vi "TPP-printer-v3.3.vi"() -> ()   [LabVIEW 2015]
uses:
  <vilib>/Math Plots/3D Math Plots/3D Scatter/3D Scatter XCtrl/3D Scatter.xctl
  <vilib>/DAQmx/write.llb/DAQmx Write (Digital Bool 1Line 1Point).vi
  SubNPC3SG.llb/device variables.vi
  <vilib>/Utility/file.llb/Read Delimited Spreadsheet (I64).vi
  <vilib>/Math Plots/3D Math Plots/3D Scatter/3D Scatter Datatype/Public/Plot Helper (Vector).vi
  <vilib>/DAQmx/create/channels.llb/DAQmx Create Channel (DO-Digital Output).vi
  <vilib>/DAQmx/miscellaneous.llb/DAQmx Fill In Error Info.vi
  <vilib>/Math Plots/3D Math Plots/3D Scatter/3D Scatter Datatype/3D Scatter Datatype.lvclass
panel:
  in  "Stopp":bool
  in  "Z轴驱动序列号":string="27002049"
  out "当前状态：":string
  in  "选项卡控件":enum32{"参数设置", "模型预览", "打印监控", "信息反馈"}(tab)
  in  "打印设置":T1={"f_objecitve(mm)"=1.8, "f_tubelens(mm)"=200.0, "f_scanlens(mm)"=50.0, "模型高/um"=2.0, "XY速度(um/s) "=0.0, "比例因子(V/°)"=1.0}
  in  "I/O 设置":T2={"matlab函数目录"=path "C:/Users/eason/Documents/GitHub/TPP-3D-printer/Matlab", "读取点阵文件"=path "C:/Users/eason/Documents/GitHub/TPP-3D-printer/Matlab/grating.txt", "DO通道：shutter控制"="Dev1/port1/line0", "AO通道：X前Y后"="Dev1/ao0:1", "Z轴驱动序列号"="27002049"}
  in  "刷新设置":bool
  out "三维散点图":refnum<class "3D Plot Datatype.lvclass">[](xcontrol)
  in  "取消打印":bool
  in  "开始打印":bool
  out "XYZG当前值/um":dbl[](array[numeric])=[-6.2105263157894735, -0.5263157894736842, 0.0, 1.0] format="%#.2g"
  out "每点耗时/ms":dbl=12.012958526611328 format="%#.0f"
  out "每行耗时/s":dbl=1.5567584037780762 format="%#.2g"
  out "每层耗时/min":dbl format="%#.2g"
  out "当前完成量：":u8(slide)=3 scale=0.0..100.0
  out "%":dbl=3.284878476249388 format="%#.2g"
  out "耗时/min":dbl=1.0008915185928344 format="%#.2g"
  in  "选项卡控件 2":enum32{"路径模拟", "PZT监控"}(tab)
  out "三维散点图 2":refnum<class "3D Plot Datatype.lvclass">[](xcontrol)
  in  "Drehschalter 2":dbl(knob) caption="2" min=-10.0 max=90.0 scale=0.0..100.0 scale format="%.3f"
  in  "Drehschalter 1":dbl(knob) caption="1" min=-10.0 max=90.0 scale=0.0..100.0 scale format="%.3f"
  in  "Drehschalter 0":dbl(knob) caption="0" min=-10.0 max=90.0 scale=0.0..100.0 scale format="%.3f"
  in  "Registerkarte":T3(tab)
  in  "Loop 2":bool caption="Loop"
  in  "Remote 2":bool caption="Remote"
  in  "Loop 1":bool caption="Loop"
  in  "Remote 1":bool caption="Remote"
  in  "Remote 0":bool caption="Remote"
  in  "Loop 0":bool caption="Loop"
  in  "Port":refnum<visa-resource-name>="COM1"
  in  "Refresh":bool
  out "Serial Number":string="RS232"
  out "Firmware Release Date":string="RS232"
  out "Version Number":string="RS232"
  out "Device":string="RS232"
  in  "com-write":bool caption="Logging"
  out "Receive Buffer":string
  out "Send Buffer":string
  in  "SendString":string caption="Enter Command"
  in  "Send":bool caption="Temp"
  in  "Clear":bool caption="Temp"
  out "Last Error":string="RS232"
  out "Last Command":string="RS232" caption="Command"
  in  "save sequence":bool caption="Loop"
  in  "load sequence":bool caption="Loop"
  in  "start sequence":bool caption="Loop"
  in  "sequence string":string
  out "时刻":T4={"点时间"=timestamp(3595558893.17812 s since 1904-01-01), "行时间"=timestamp(3595558891.757594 s since 1904-01-01), "层时间"=timestamp(3595558833.124629 s since 1904-01-01)}
  out "起始时间":timestamp
  out "暂停时间/min":dbl=1.0008915185928344 format="%#.2g"
  out "当前扫描速度(um/s)":dbl
  in  "dc level 3 out":refnum<vi>
  in  "dc level 2 out":refnum<vi>
  in  "dc level 1 out":refnum<vi>
  in  "dc level 1 in":refnum<vi>
  in  "dc level 2 in":refnum<vi>
  in  "dc level 3 in":refnum<vi>
  in  "loop 1 in":refnum<vi>
  in  "loop 2 in":refnum<vi>
  in  "loop 3 in":refnum<vi>
  in  "command in":refnum<vi>
  out "XYZG坐标表":dbl[][](array[numeric])
  # "Piezo 1"
  # "Piezo 2"
  # "Piezo 3"
  # "Loop"
  # "Remote"
  # "possible commands in sequence\n\nset,1,2.34 (actuator position)\nwait,5  - (holding time in sec.)\nstop - (terminate sequence)\n\nexample:\nset,1,2.134\nwait,5\nset,0,22.66\nwait,10\nstop"
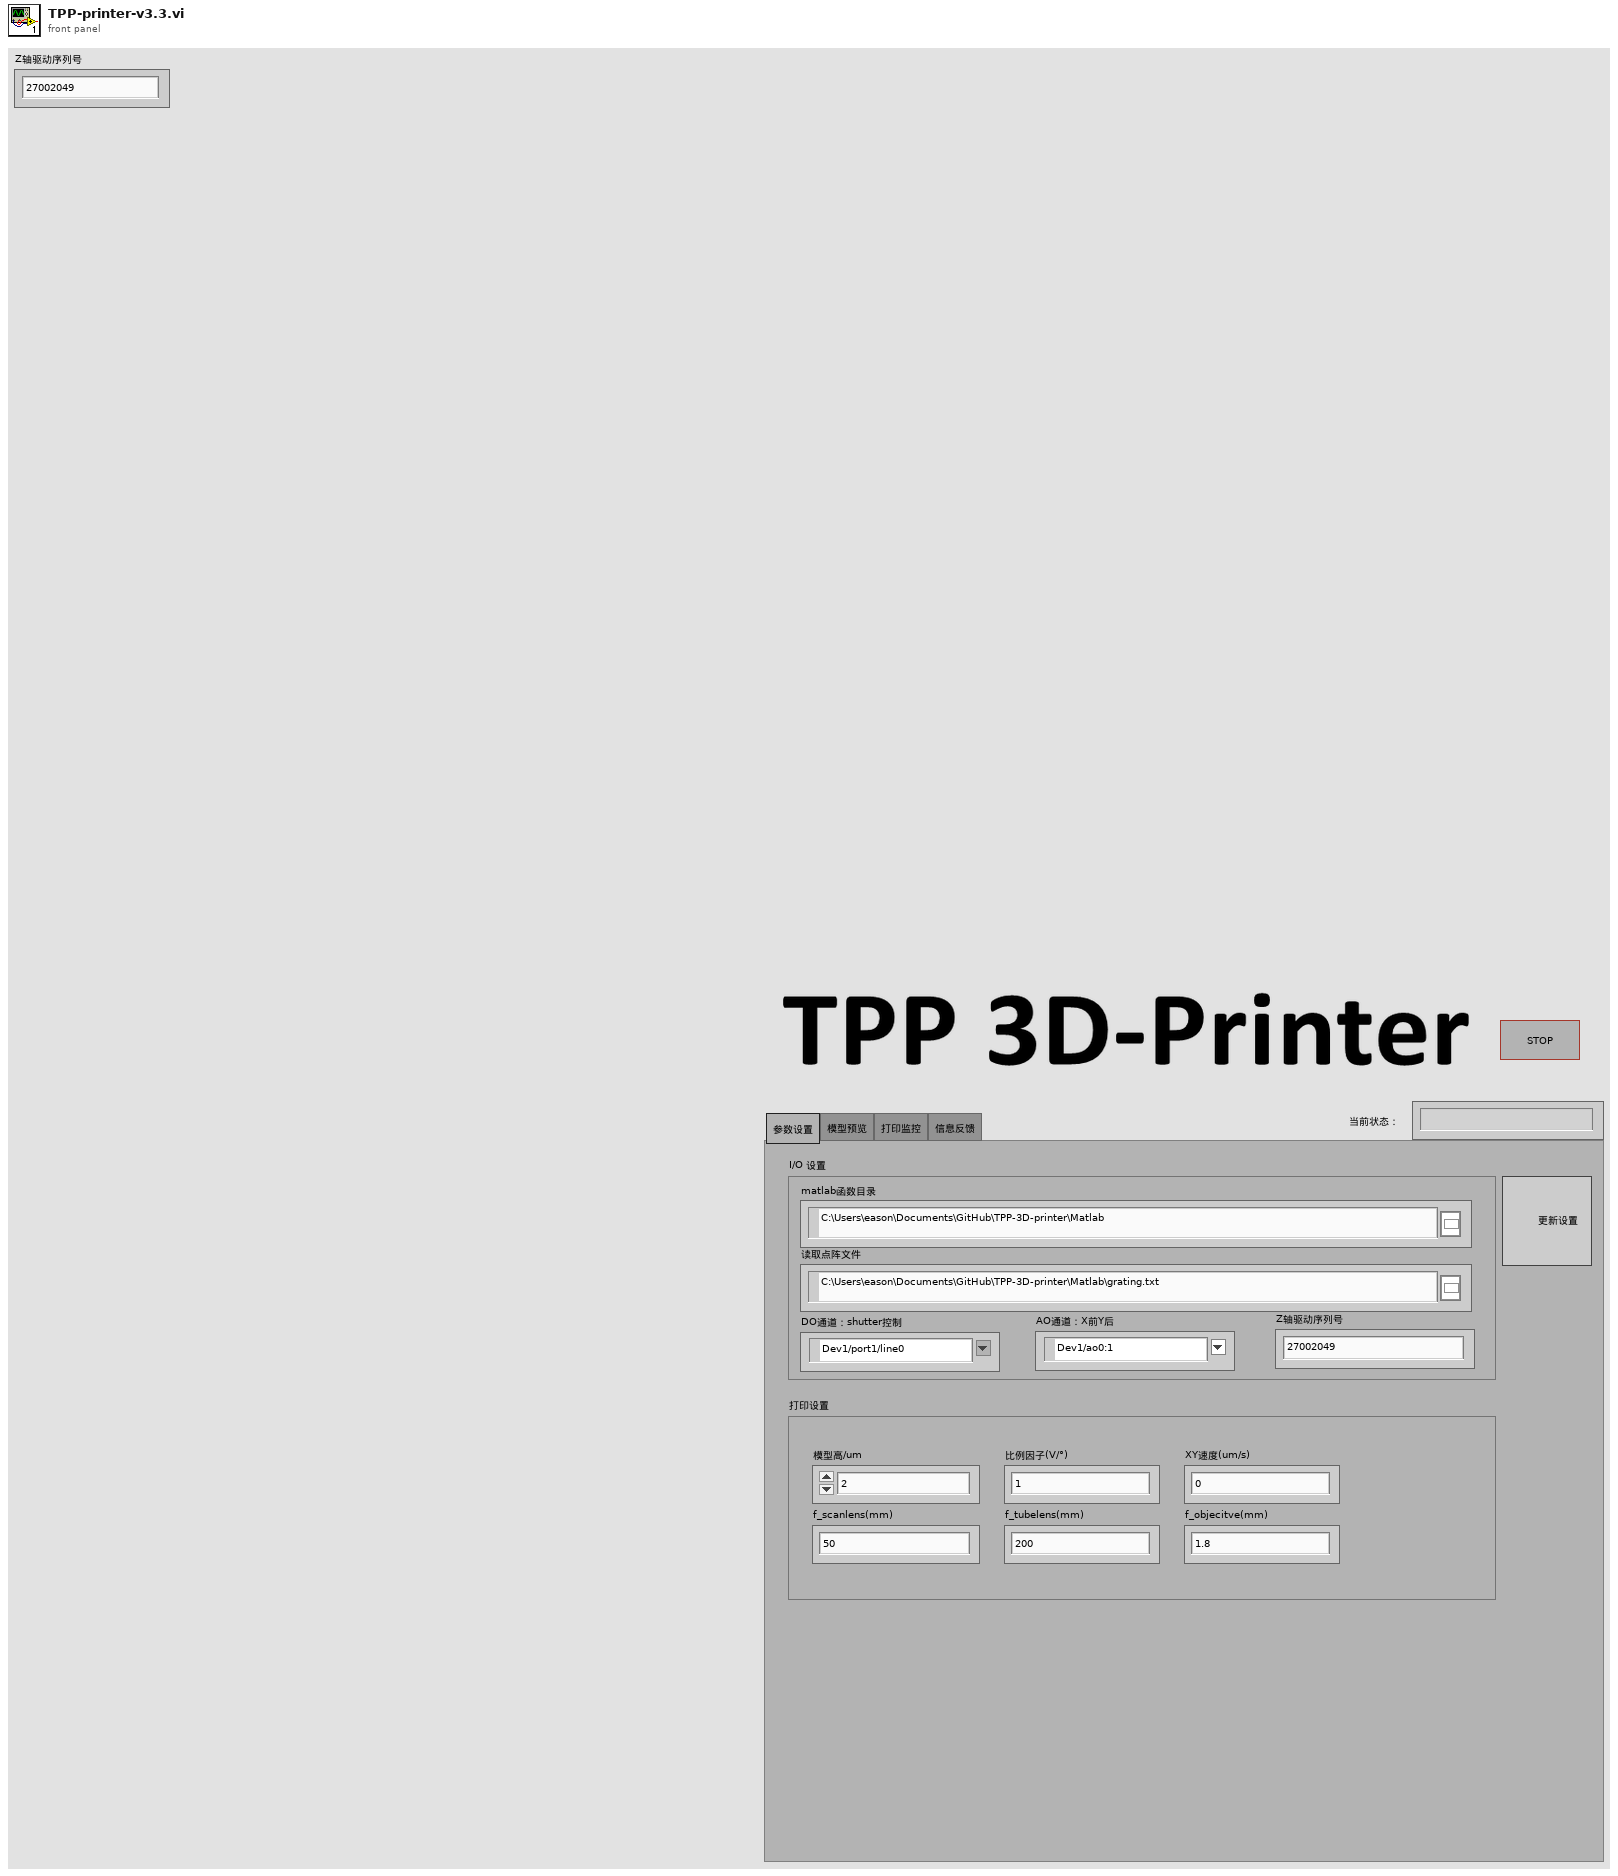
[diagram p1: front panel]
types:
  T1 = cluster{"f_objecitve(mm)":dbl, "f_tubelens(mm)":dbl, "f_scanlens(mm)":dbl, "模型高/um":dbl, "XY速度(um/s) ":dbl, "比例因子(V/°)":dbl}
  T2 = cluster{"matlab函数目录":path, "读取点阵文件":path, "DO通道：shutter控制":tag, "AO通道：X前Y后":tag, "Z轴驱动序列号":string}
  T3 = enum32{"Settings", "Info", "Communication", "Sequence"}
  T4 = cluster{"点时间":timestamp, "行时间":timestamp, "层时间":timestamp}
  T5 = enum16{"open", "replace", "create", "open or create", "replace or create", "replace or create with confirmation"}
  T6 = cluster{"Registerkarte":refnum<vi>, "Array IsActor":bool[], "Array loop":bool[], "Array remote":bool[]}
  T7 = cluster{"Array dc-level":dbl[], "VAR Temp":string, "VAR USB":string, "Array IsActor":bool[], "Array actor-name":string[], "Array axis":string[], "Array loop":bool[], "Array remote":bool[], "Array ovl":bool[]}
  T8 = cluster{"Drehschalter 0":refnum<vi>, "Drehschalter 1":refnum<vi>, "Drehschalter 2":refnum<vi>, "Array loop":bool[], "Array IsActor":bool[], "Array clmin":dbl[], "Array clmax":dbl[], "VAR Vmin":dbl, "VAR Vmax":dbl, "Array dc-level open":dbl[], "Array dc-level closed":dbl[], "VAR actualisation":bool}
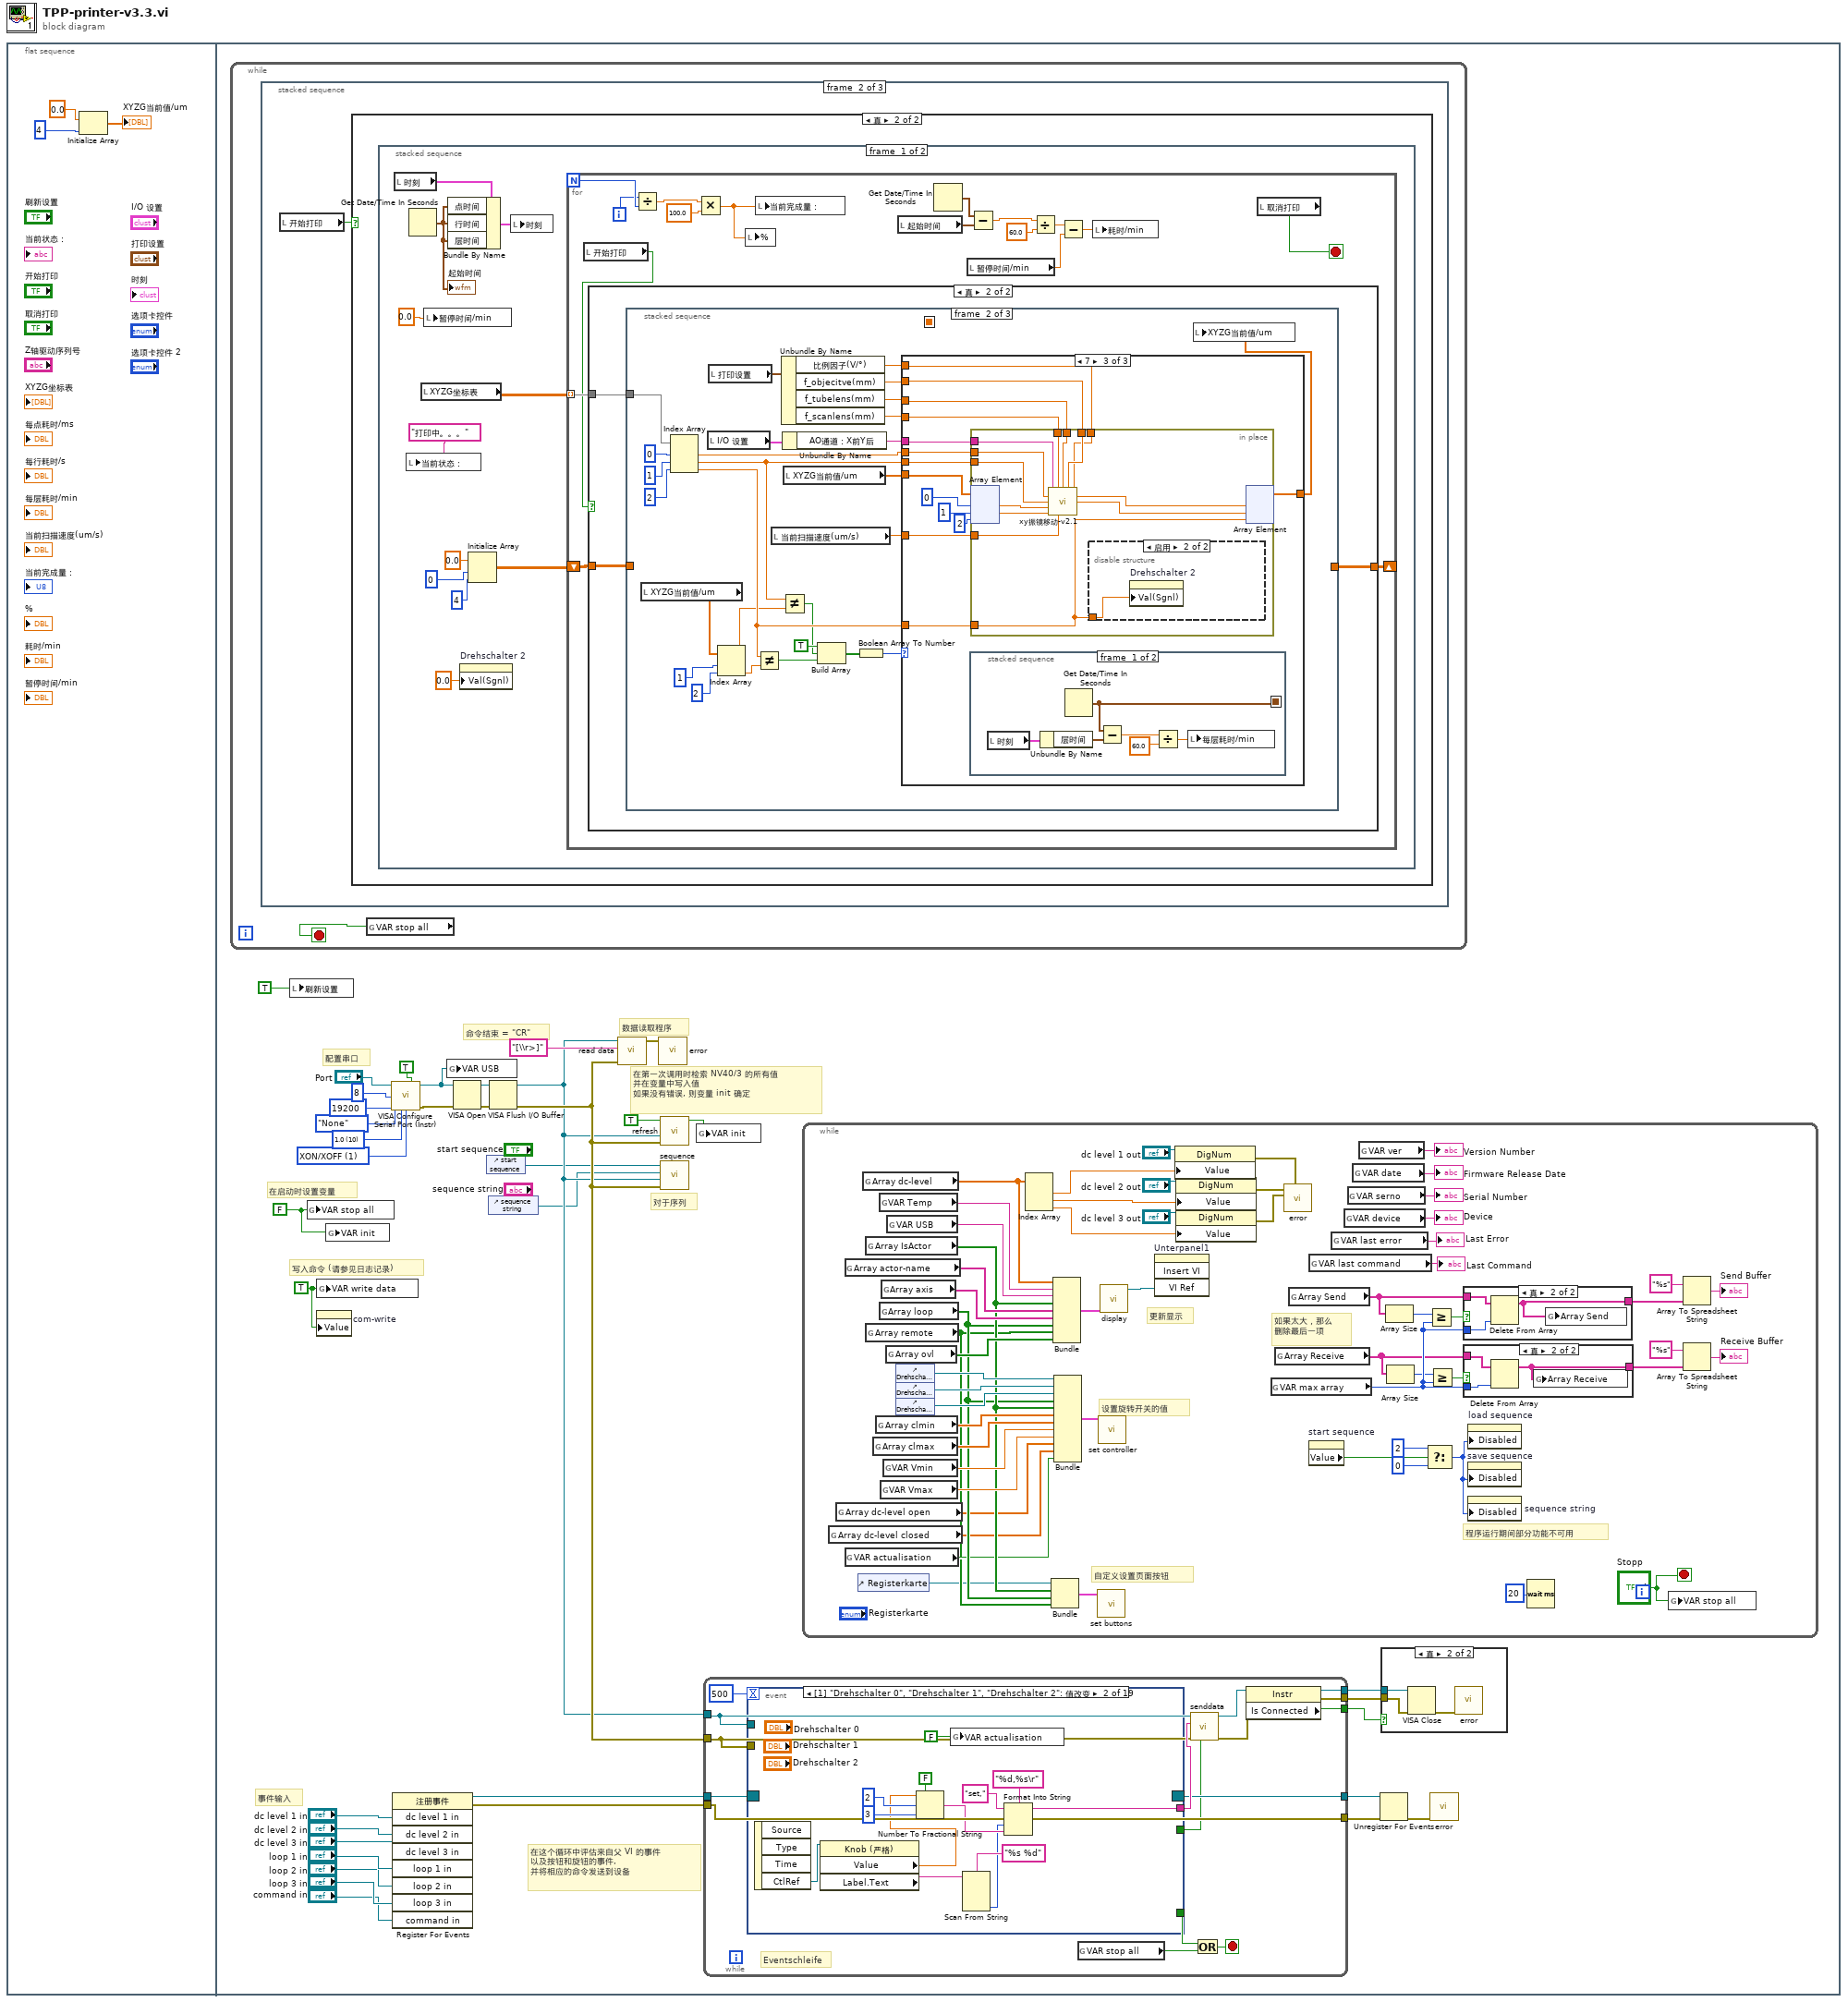
[diagram p0: block diagram]
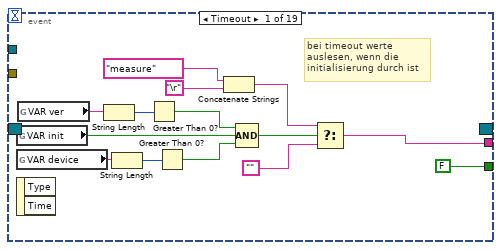
[diagram p3: hidden frame]
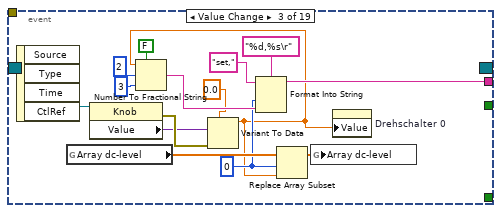
[diagram p4: hidden frame]
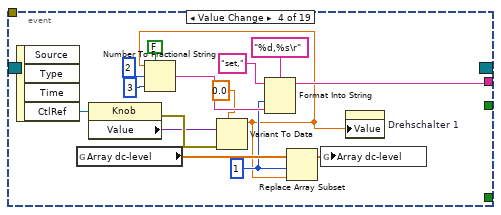
[diagram p5: hidden frame]
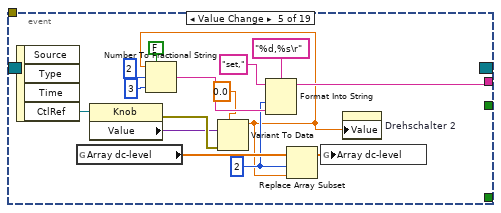
[diagram p6: hidden frame]
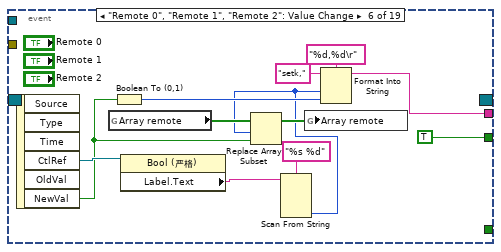
[diagram p7: hidden frame]
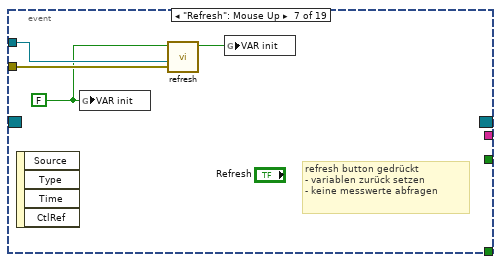
[diagram p8: hidden frame]
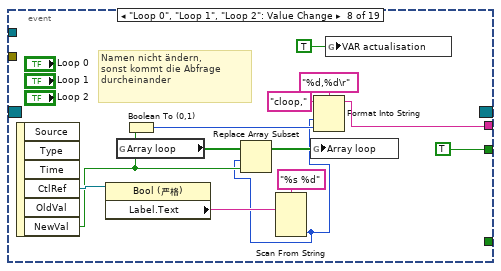
[diagram p9: hidden frame]
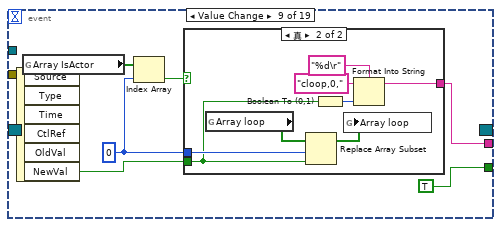
[diagram p10: hidden frame]
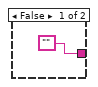
[diagram p11: hidden frame]
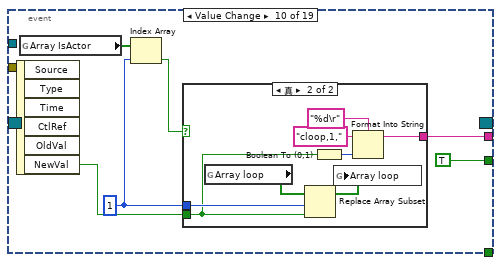
[diagram p12: hidden frame]
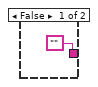
[diagram p13: hidden frame]
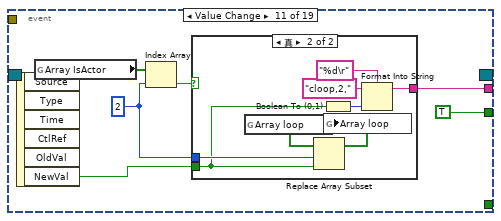
[diagram p14: hidden frame]
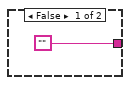
[diagram p15: hidden frame]
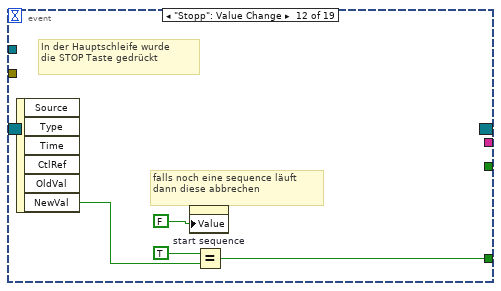
[diagram p16: hidden frame]
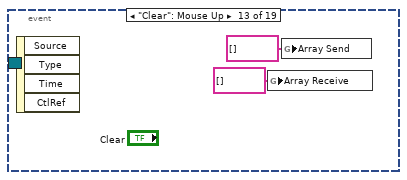
[diagram p17: hidden frame]
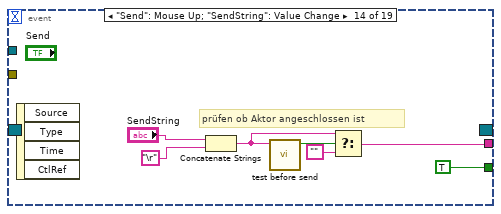
[diagram p18: hidden frame]
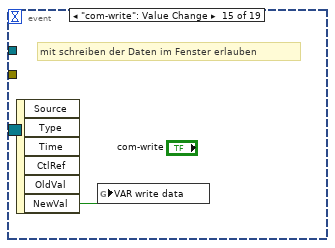
[diagram p19: hidden frame]
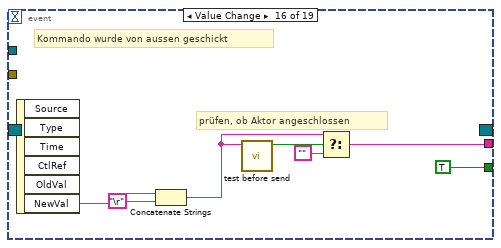
[diagram p20: hidden frame]
diagram:
  n1 = flat-sequence {
    frame #0 {
      n2 = Initialize Array(0.0 ("元素"), 4 ("维数大小")) -> (→"XYZG当前值/um":dbl[])
    }
    frame #1 {
      w12 = TRUE ("VAR write data")
      w16 = FALSE ("VAR ovl 3")
      w13 = u16 1 items=["Kein", "XON/XOFF", "RTS/CTS", "XON/XOFF & RTS/CTS", "DTR/DSR", "XON/XOFF & DTR/DSR"] ("flow control (0:none)")
      w32 = u16 10 items=["1.0"=10, "1.5"=15, "2.0"=20] ("stop bits (10: 1 bit)")
      # "对于序列"
      # "写入命令 (请参见日志记录)"
      # "命令结束 = \"CR\""
      # "数据读取程序"
      # "在第一次调用时检索 NV40/3 的所有值\n并在变量中写入值\n如果没有错误, 则变量 init 确定"
      # "在启动时设置变量"
      # "配置串口"
      # "事件输入"
      # "在这个循环中评估来自父 VI 的事件\n以及按钮和旋钮的事件, \n并将相应的命令发送到设备"
      n3 = while {
        stop <- w336 stop-if-true
        n4 = stacked-sequence {
          frame #0 {
            n5 = local read "刷新设置"() -> (w337:bool)
            n6 = case shown="真" w337 {
              frame False {
              }
              frame True {
                w344 = 0.0 ("每点耗时/ms")
                w353 = 0.0 ("速度(°/s)")
                # "平移坐标中心至X0Y0"
                n7 = local read "I/O 设置"() -> (w368:T2)
                n8 = local write "每点耗时/ms"(w344) -> ()
                n9 = local write "每行耗时/s"(w344) -> ()
                n10 = local write "每层耗时/min"(w344) -> ()
                n11 = disable-structure shown="禁用" {
                  disable-tunnel: w344 -> [w373 _]
                  frame Disabled {
                    n12 = local read "I/O 设置"() -> (w371:T2)
                    n13 = Unbundle By Name(w371) -> ("Z轴驱动序列号"=w370:string)
                    n14 = call "z物镜移动.vi"("position"=w373, "maxVelocity"=5.0, "SerialNumber"=w370) -> ()  [unwired: 6 in, 3 out]
                  }
                  frame Enabled {
                  }
                }
                n15 = Unbundle By Name(w368) -> ("matlab函数目录"=w366:path, "读取点阵文件"=w367:path)
                n16 = local read "打印设置"() -> (w365:T1)
                n17 = Unbundle By Name(w365) -> ("模型高/um"=w364:dbl)
                n18 = call-poly <vilib>:"Read Delimited Spreadsheet.vi"("file path (dialog if empty)"=w367) -> ("all rows"=w369:i64[][])  [unwired: 9 in, 5 out]
                n19 = script code="addpath(add_path);\ncol_x=2;\ncol_y=3;\ncol_z=4;\nxyzg=path_generation( in,col_x,col_y,col_z,z_length );"("in"=w369, "z_length"=w364, "add_path"=w366) -> ("xyzg"=w354:dbl[][])  [unwired: 1 in, 1 out]
                n20 = local read "打印设置"() -> (w350:T1)
                n21 = local read "I/O 设置"() -> (w352:T2)
                n22 = Unbundle By Name(w352) -> ("AO通道：X前Y后"=w351:tag)
                n23 = Unbundle By Name(w350) -> ("比例因子(V/°)"=w343:dbl, "f_objecitve(mm)"=w347:dbl, "f_tubelens(mm)"=w348:dbl, "f_scanlens(mm)"=w349:dbl)
                n24 = call "xy振镜移动-v2.1.vi"("AO通道：X前Y后"=w351, "f_scanlens(mm)"=w349, "f_tubelens(mm)"=w348, "f_objecitve(mm)"=w347, "比例因子(V/°)"=w343, "x终止位(um)"=w353, "y终止位(um)"=w353, "速度(um/s)"=w353) -> ()  [unwired: 6 in, 2 out]
                n25 = local write "XYZG坐标表"(w354) -> ()
                n26 = Array Max & Min(array=w354) -> (max value=w356:dbl, min value=w357:dbl)  [unwired: 2 out]
                n27 = Subtract(x=w356, y=w357) -> (x-y=w355:dbl)
                n28 = Index Array(array=w354, index (col) #1=0 ("禁用的索引 (列)"), index (col) #2=1 ("索引 (列)"), index (col) #3=2 ("索引 (列)")) -> (element #1=w360:dbl[], element #2=w359:dbl[], element #3=w358:dbl[])  [unwired: 3 in]
                n29 = local write "刷新设置"(FALSE ("刷新设置")) -> ()
                n30 = Divide(x=w360, y=w355) -> (x/y=w339:dbl[])
                n31 = Divide(x=w359, y=w355) -> (x/y=w338:dbl[])
                n32 = Divide(x=w358, y=w355) -> (x/y=w340:dbl[])
                n33 = local write "当前状态："("初始化。。。" ("当前状态：")) -> ()
                n34 = call-poly <vilib>:"Plot Helper.vi"("z vector"=w340, "y vector"=w338, "x vector"=w339) -> ("error out"=w341:errorcluster, "3D Plot lvclass Array out"=→"三维散点图":refnum<class "3D Plot Datatype.lvclass">[])  [unwired: 3 in, 4 out]
                n35 = call <vilib>:"Simple Error Handler.vi"("error in (no error)"=w341) -> ()  [unwired: 4 in, 5 out]
              }
            }
          }
          frame #1 {
            n36 = local read "开始打印"() -> (w374:bool)
            n37 = case shown="真" w374 {
              frame False {
              }
              frame True {
                n38 = stacked-sequence {
                  frame #0 {
                    n39 = local read "时刻"() -> (w382:T4)
                    n40 = local write "当前状态："("打印中。。。" ("当前状态：")) -> ()
                    n41 = Get Date/Time In Seconds() -> (seconds since 1Jan1904=w381:timestamp)
                    "起始时间" <- w381
                    n42 = local read "XYZG坐标表"() -> (w384:dbl[][])
                    n43 = local write "暂停时间/min"(0.0 ("暂停耗时/min")) -> ()
                    n44 = Bundle By Name(cluster=w382, "点时间"=w381, "行时间"=w381, "层时间"=w381) -> (w380:T4)
                    n45 = property on="Drehschalter 2" class="Knob (严格)"("Val(Sgnl)"=0.0 ("值(信号)")) -> ()  [unwired: 2 in, 2 out]
                    n46 = Initialize Array(0.0 ("元素"), 0 ("维数大小"), 4 ("维数大小")) -> (w378:dbl[][])
                    n47 = local write "时刻"(w380) -> ()
                    n48 = for {
                      N -> [w401]
                      tunnel: w384 -> [w402] mode=indexing
                      shift-right: [w387] -> _
                      shift-left: w378 -> [w388]
                      i -> [w386]
                      stop <- w397 stop-if-true
                      n49 = local read "开始打印"() -> (w398:bool)
                      n50 = case shown="真" w398 {
                        tunnel: w402 -> [_ w421]
                        tunnel: w388 -> [w403 w420]
                        tunnel: [w403 w419] -> w387
                        frame False {
                          n51 = stacked-sequence {
                            seq-local: [w404 _ _] -> [_ _ w412]
                            frame #0 {
                              n52 = Get Date/Time In Seconds() -> (seconds since 1Jan1904=w404:timestamp)
                            }
                            frame #1 {
                              n53 = while {
                                stop <- w406 stop-if-true
                                n54 = local read "开始打印"() -> (w408:bool)
                                n55 = local read "取消打印"() -> (w407:bool)
                                n56 = Or(x=w408, y=w407) -> (x .or. y?=w406:bool)
                              }
                              n57 = local write "当前状态："("暂停打印" ("当前状态：")) -> ()
                            }
                            frame #2 {
                              n58 = Get Date/Time In Seconds() -> (seconds since 1Jan1904=w409:timestamp)
                              n59 = local read "时刻"() -> (w411:T4)
                              n60 = Subtract(x=w409, y=w412) -> (x-y=w417:dbl)
                              n61 = Bundle By Name(cluster=w411, "点时间"=w409, "行时间"=w409, "层时间"=w409) -> (w410:T4)
                              n62 = local read "暂停时间/min"() -> (w414:dbl)
                              n63 = Divide(x=w417, y=60.0) -> (x/y=w415:dbl)
                              n64 = local write "时刻"(w410) -> ()
                              n65 = Add(x=w415, y=w414) -> (x+y=w413:dbl)
                              n66 = local write "暂停时间/min"(w413) -> ()
                              n67 = local write "当前状态："("打印中。。。" ("当前状态：")) -> ()
                            }
                          }
                        }
                        frame True {
                          n68 = stacked-sequence {
                            seq-local: [w423 _ _] -> [_ _ w595]
                            tunnel: w421 -> [w422 w469 _]
                            tunnel: w420 -> [_ _ w594]
                            tunnel: [_ _ w592] -> w419
                            frame #0 {
                              n69 = local read "XYZG当前值/um"() -> (w426:dbl[])
                              n70 = Index Array(array=w426, index=3 ("索引")) -> (element=w424:dbl)
                              n71 = Index Array(array=w422, index=3 ("禁用的索引 (列)")) -> (element=w423:dbl)
                              n72 = Not Equal?(x=w424, y=w423) -> (x != y?=w427:bool)
                              n73 = case shown="真" w427 {
                                tunnel: w423 -> [_ w430]
                                frame False {
                                }
                                frame True {
                                n74 = case shown="1" w430 {
                                frame 0, Default {
                                # "1，关闭shutter"
                                n75 = local read "I/O 设置"() -> (w434:T2)
                                n76 = Unbundle By Name(w434) -> ("DO通道：shutter控制"=w433:tag)
                                n77 = call-poly <vilib>:"DAQmx Create Virtual Channel.vi"("lines"=w433) -> ("task out"=w445:refnum<k21>, "error out"=w444:errorcluster)  [unwired: 13 in]
                                n78 = local write "当前扫描速度(um/s)"(0.0 ("扫描速度(°/s)")) -> ()
                                n79 = call-poly <vilib>:"DAQmx Write.vi"("task/channels in"=w445, "data"=FALSE, "error in"=w444) -> ("task out"=w442:refnum<k21>, "error out"=w441:errorcluster)  [unwired: 10 in, 1 out]
                                n80 = call <vilib>:"DAQmx Start Task.vi"("task/channels in"=w442, "error in"=w441) -> ("task out"=w436:refnum<k21>, "error out"=w435:errorcluster)  [unwired: 12 in]
                                n81 = call <vilib>:"DAQmx Stop Task.vi"("task/channels in"=w436, "error in"=w435) -> ("task out"=w440:refnum<k21>, "error out"=w439:errorcluster)  [unwired: 12 in]
                                n82 = call <vilib>:"DAQmx Clear Task.vi"("task in"=w440, "error in"=w439) -> ("error out"=w438:errorcluster)  [unwired: 13 in]
                                n83 = call <vilib>:"Simple Error Handler.vi"("error in (no error)"=w438) -> ()  [unwired: 4 in, 5 out]
                                }
                                frame 1 {
                                # "1，打开shutter\n2，设定速度（斜率）\n3，等待"
                                n84 = stacked-sequence {
                                frame #0 {
                                n85 = local read "I/O 设置"() -> (w449:T2)
                                n86 = Unbundle By Name(w449) -> ("DO通道：shutter控制"=w448:tag)
                                n87 = call-poly <vilib>:"DAQmx Create Virtual Channel.vi"("lines"=w448) -> ("task out"=w459:refnum<k21>, "error out"=w458:errorcluster)  [unwired: 13 in]
                                n88 = call-poly <vilib>:"DAQmx Write.vi"("task/channels in"=w459, "data"=TRUE, "error in"=w458) -> ("task out"=w456:refnum<k21>, "error out"=w455:errorcluster)  [unwired: 10 in, 1 out]
                                n89 = call <vilib>:"DAQmx Start Task.vi"("task/channels in"=w456, "error in"=w455) -> ("task out"=w451:refnum<k21>, "error out"=w450:errorcluster)  [unwired: 12 in]
                                n90 = call <vilib>:"DAQmx Stop Task.vi"("task/channels in"=w451, "error in"=w450) -> ("task out"=w454:refnum<k21>, "error out"=w453:errorcluster)  [unwired: 12 in]
                                n91 = call <vilib>:"DAQmx Clear Task.vi"("task in"=w454, "error in"=w453) -> ("error out"=w452:errorcluster)  [unwired: 13 in]
                                n92 = call <vilib>:"Simple Error Handler.vi"("error in (no error)"=w452) -> ()  [unwired: 4 in, 5 out]
                                }
                                frame #1 {
                                n93 = Wait (ms)(milliseconds to wait=u32 0 ("等待时间（毫秒）")) -> ()  [unwired: 1 out]
                                }
                                }
                                n94 = local read "打印设置"() -> (w447:T1)
                                n95 = Unbundle By Name(w447) -> ("XY速度(um/s)"=w446:dbl)
                                n96 = local write "当前扫描速度(um/s)"(w446) -> ()
                                }
                                }
                                n97 = local read "XYZG当前值/um"() -> (w432:dbl[])
                                n98 = Replace Array Subset(array=w432, new element=w430, index=3 ("索引")) -> (w429:dbl[])
                                n99 = local write "XYZG当前值/um"(w429) -> ()
                                }
                              }
                            }
                            frame #1 {
                              n100 = local read "XYZG当前值/um"() -> (w477:dbl[])
                              n101 = Index Array(array=w469, index #1=0 ("禁用的索引 (列)"), index #2=1 ("索引"), index #3=2 ("索引")) -> (element #1=w481:dbl, element #2=w472:dbl, element #3=w476:dbl)
                              n102 = local read "I/O 设置"() -> (w463:T2)
                              n103 = local read "打印设置"() -> (w468:T1)
                              n104 = Index Array(array=w477, index #1=1 ("索引"), index #2=2 ("索引")) -> (element #1=w471:dbl, element #2=w473:dbl)
                              n105 = Not Equal?(x=w476, y=w473) -> (x != y?=w475:bool)
                              n106 = local read "当前扫描速度(um/s)"() -> (w486:dbl)
                              n107 = Not Equal?(x=w472, y=w471) -> (x != y?=w470:bool)
                              n108 = Unbundle By Name(w468) -> ("比例因子(V/°)"=w467:dbl, "f_objecitve(mm)"=w465:dbl, "f_tubelens(mm)"=w466:dbl, "f_scanlens(mm)"=w464:dbl)
                              n109 = Unbundle By Name(w463) -> ("AO通道：X前Y后"=w462:tag)
                              n110 = local read "XYZG当前值/um"() -> (w484:dbl[])
                              n111 = Build Array(TRUE ("元素"), w470, w475) -> (w483:bool[])
                              n112 = Boolean Array To Number(Boolean array=w483) -> (number=w461:u32)
                              n113 = case shown="7" w461 {
                                tunnel: w462 -> [w493 w525 w561]
                                tunnel: w481 -> [w495 w526 w560]
                                tunnel: w484 -> [w498 w527 w559]
                                tunnel: [w489 w520 w551] -> w485
                                tunnel: w486 -> [w494 w528 w558]
                                tunnel: w472 -> [_ w524 w557]
                                tunnel: w476 -> [_ _ w552]
                                tunnel: w464 -> [w492 w523 w556]
                                tunnel: w466 -> [w491 w522 w555]
                                tunnel: w465 -> [w490 w521 w554]
                                tunnel: w467 -> [w488 w519 w550]
                                frame 1, Default {
                                n114 = stacked-sequence {
                                seq-local: [w501 _] -> [_ w507]
                                frame #0 {
                                n115 = local read "时刻"() -> (w499:T4)
                                n116 = Unbundle By Name(w499) -> ("点时间"=w500:timestamp)
                                n117 = Get Date/Time In Seconds() -> (seconds since 1Jan1904=w501:timestamp)
                                n118 = Subtract(x=w501, y=w500) -> (x-y=w504:dbl)
                                n119 = Multiply(x=w504, y=1000.0) -> (x*y=w502:dbl)
                                n120 = local write "每点耗时/ms"(w502) -> ()
                                }
                                frame #1 {
                                n121 = local read "时刻"() -> (w505:T4)
                                n122 = Bundle By Name(cluster=w505, "点时间"=w507) -> (w506:T4)
                                n123 = local write "时刻"(w506) -> ()
                                }
                                }
                                n124 = in-place {
                                in-place-border: w495 -> [w513]
                                in-place-border: w494 -> [w518]
                                in-place-border: w493 -> [w517]
                                in-place-border: w492 -> [w516]
                                in-place-border: w491 -> [w515]
                                in-place-border: w490 -> [w514]
                                in-place-border: w488 -> [w508]
                                n125 = in-place-array #1(w498, 0, 1) -> (w512:dbl, w511:dbl)
                                n126 = call "xy振镜移动-v2.1.vi"("AO通道：X前Y后"=w517, "f_scanlens(mm)"=w516, "f_tubelens(mm)"=w515, "f_objecitve(mm)"=w514, "比例因子(V/°)"=w508, "x终止位(um)"=w513, "y终止位(um)"=w511, "x初始位(um)"=w512, "y初始位(um)"=w511, "速度(um/s)"=w518) -> ("x终止位(um) 2"=w510:dbl, "y终止位(um) 2"=w509:dbl)  [unwired: 4 in]
                                n127 = in-place-array #1(w510, w509) -> (w489:dbl[])  [unwired: 2 out]
                                }
                                }
                                frame 3 {
                                n128 = in-place {
                                in-place-border: w526 -> [w549]
                                in-place-border: w528 -> [w548]
                                in-place-border: w525 -> [w547]
                                in-place-border: w524 -> [w543]
                                in-place-border: w523 -> [w546]
                                in-place-border: w522 -> [w545]
                                in-place-border: w521 -> [w544]
                                in-place-border: w519 -> [w538]
                                n129 = in-place-array #2(w527, 0, 1) -> (w542:dbl, w541:dbl)
                                n130 = call "xy振镜移动-v2.1.vi"("AO通道：X前Y后"=w547, "f_scanlens(mm)"=w546, "f_tubelens(mm)"=w545, "f_objecitve(mm)"=w544, "比例因子(V/°)"=w538, "x终止位(um)"=w549, "y终止位(um)"=w543, "x初始位(um)"=w542, "y初始位(um)"=w541, "速度(um/s)"=w548) -> ("x终止位(um) 2"=w540:dbl, "y终止位(um) 2"=w539:dbl)  [unwired: 4 in]
                                n131 = in-place-array #2(w540, w539) -> (w520:dbl[])  [unwired: 2 out]
                                }
                                n132 = stacked-sequence {
                                seq-local: [w533 _] -> [_ w537]
                                frame #0 {
                                n133 = local read "时刻"() -> (w531:T4)
                                n134 = Unbundle By Name(w531) -> ("行时间"=w532:timestamp)
                                n135 = Get Date/Time In Seconds() -> (seconds since 1Jan1904=w533:timestamp)
                                n136 = Subtract(x=w533, y=w532) -> (x-y=w534:dbl)
                                n137 = local write "每行耗时/s"(w534) -> ()
                                }
                                frame #1 {
                                n138 = local read "时刻"() -> (w535:T4)
                                n139 = Bundle By Name(cluster=w535, "行时间"=w537) -> (w536:T4)
                                n140 = local write "时刻"(w536) -> ()
                                }
                                }
                                }
                                frame 7 {
                                n141 = stacked-sequence {
                                seq-local: [w569 _] -> [_ w572]
                                frame #0 {
                                n142 = local read "时刻"() -> (w564:T4)
                                n143 = Unbundle By Name(w564) -> ("层时间"=w565:timestamp)
                                n144 = Get Date/Time In Seconds() -> (seconds since 1Jan1904=w569:timestamp)
                                n145 = Subtract(x=w569, y=w565) -> (x-y=w568:dbl)
                                n146 = Divide(x=w568, y=60.0) -> (x/y=w566:dbl)
                                n147 = local write "每层耗时/min"(w566) -> ()
                                }
                                frame #1 {
                                n148 = local read "时刻"() -> (w571:T4)
                                n149 = Bundle By Name(cluster=w571, "层时间"=w572) -> (w570:T4)
                                n150 = local write "时刻"(w570) -> ()
                                }
                                }
                                n151 = in-place {
                                in-place-border: w560 -> [w584]
                                in-place-border: w558 -> [w575]
                                in-place-border: w561 -> [w585]
                                in-place-border: w557 -> [w583]
                                in-place-border: w556 -> [w578]
                                in-place-border: w555 -> [w577]
                                in-place-border: w554 -> [w576]
                                in-place-border: w552 -> [w573]
                                in-place-border: w550 -> [w574]
                                n152 = in-place-array #3(w559, 0, 1, 2) -> (w580:dbl, w579:dbl)  [unwired: 1 out]
                                n153 = call "xy振镜移动-v2.1.vi"("AO通道：X前Y后"=w585, "f_scanlens(mm)"=w578, "f_tubelens(mm)"=w577, "f_objecitve(mm)"=w576, "比例因子(V/°)"=w574, "x终止位(um)"=w584, "y终止位(um)"=w583, "x初始位(um)"=w580, "y初始位(um)"=w579, "速度(um/s)"=w575) -> ("x终止位(um) 2"=w582:dbl, "y终止位(um) 2"=w581:dbl)  [unwired: 4 in]
                                n154 = disable-structure shown="启用" {
                                disable-tunnel: w573 -> [w589 w590]
                                frame Disabled {
                                n155 = local read "I/O 设置"() -> (w587:T2)
                                n156 = Unbundle By Name(w587) -> ("Z轴驱动序列号"=w586:string)
                                n157 = call "z物镜移动.vi"("position"=w589, "maxVelocity"=5.0, "SerialNumber"=w586) -> ()  [unwired: 6 in, 3 out]
                                }
                                frame Enabled {
                                n158 = property on="Drehschalter 2" class="Knob (严格)"("Val(Sgnl)"=w590) -> ()  [unwired: 2 in, 2 out]
                                }
                                }
                                n159 = in-place-array #3(w582, w581, w573) -> (w551:dbl[])  [unwired: 3 out]
                                }
                                }
                              }
                              n160 = local write "XYZG当前值/um"(w485) -> ()
                            }
                            frame #2 {
                              n161 = local read "XYZG当前值/um"() -> (w593:dbl[])
                              n162 = local read "选项卡控件 2"() -> (w591:enum32{"路径模拟", "PZT监控"})
                              n163 = Insert Into Array(array=w594, new element=w593) -> (w592:dbl[][])  [unwired: 2 in]
                              n164 = case shown="\"路径模拟\", 默认" w591 {
                                tunnel: w592 -> [w596 _]
                                frame "路径模拟", Default {
                                n165 = Index Array(array=w596, index (col) #1=0 ("禁用的索引 (列)"), index (col) #2=1 ("索引 (列)"), index (col) #3=2 ("索引 (列)")) -> (element #1=w600:dbl[], element #2=w599:dbl[], element #3=w598:dbl[])  [unwired: 3 in]
                                n166 = call-poly <vilib>:"Plot Helper.vi"("z vector"=w598, "y vector"=w599, "x vector"=w600) -> ("error out"=w597:errorcluster, "3D Plot lvclass Array out"=→"三维散点图 2":refnum<class "3D Plot Datatype.lvclass">[])  [unwired: 3 in, 4 out]
                                n167 = call <vilib>:"Simple Error Handler.vi"("error in (no error)"=w597) -> ()  [unwired: 4 in, 5 out]
                                }
                                frame "PZT监控" {
                                }
                              }
                              n168 = case shown="1" w595 {
                                frame 0, Default {
                                n169 = Wait (ms)(milliseconds to wait=u32 0 ("等待时间（毫秒）")) -> ()  [unwired: 1 out]
                                }
                                frame 1 {
                                # "等待"
                                n170 = Wait (ms)(milliseconds to wait=u32 0 ("等待时间（毫秒）")) -> ()  [unwired: 1 out]
                                }
                              }
                            }
                          }
                        }
                      }
                      n171 = Divide(x=w386, y=w401) -> (x/y=w400:dbl)
                      n172 = Multiply(x=w400, y=100.0) -> (x*y=w396:dbl)
                      n173 = local write "%"(w396) -> ()
                      n174 = local write "当前完成量："(w396) -> ()
                      n175 = local read "起始时间"() -> (w392:timestamp)
                      n176 = Get Date/Time In Seconds() -> (seconds since 1Jan1904=w393:timestamp)
                      n177 = local read "暂停时间/min"() -> (w390:dbl)
                      n178 = Subtract(x=w393, y=w392) -> (x-y=w395:dbl)
                      n179 = Divide(x=w395, y=60.0) -> (x/y=w391:dbl)
                      n180 = Subtract(x=w391, y=w390) -> (x-y=w389:dbl)
                      n181 = local write "耗时/min"(w389) -> ()
                      n182 = local read "取消打印"() -> (w397:bool)
                    }
                  }
                  frame #1 {
                    n183 = local read "I/O 设置"() -> (w608:T2)
                    n184 = Unbundle By Name(w608) -> ("DO通道：shutter控制"=w607:tag)
                    n185 = local write "开始打印"(FALSE ("取消打印")) -> ()
                    n186 = local write "取消打印"(FALSE ("开始打印")) -> ()
                    n187 = call-poly <vilib>:"DAQmx Create Virtual Channel.vi"("lines"=w607) -> ("task out"=w611:refnum<k21>, "error out"=w612:errorcluster)  [unwired: 13 in]
                    n188 = call-poly <vilib>:"DAQmx Write.vi"("task/channels in"=w611, "data"=FALSE, "error in"=w612) -> ("task out"=w614:refnum<k21>, "error out"=w615:errorcluster)  [unwired: 10 in, 1 out]
                    n189 = call <vilib>:"DAQmx Start Task.vi"("task/channels in"=w614, "error in"=w615) -> ("task out"=w619:refnum<k21>, "error out"=w620:errorcluster)  [unwired: 12 in]
                    n190 = call <vilib>:"DAQmx Stop Task.vi"("task/channels in"=w619, "error in"=w620) -> ("task out"=w616:refnum<k21>, "error out"=w617:errorcluster)  [unwired: 12 in]
                    n191 = call <vilib>:"DAQmx Clear Task.vi"("task in"=w616, "error in"=w617) -> ("error out"=w618:errorcluster)  [unwired: 13 in]
                    n192 = call <vilib>:"Simple Error Handler.vi"("error in (no error)"=w618) -> ()  [unwired: 4 in, 5 out]
                  }
                }
              }
            }
          }
          frame #2 {
            n193 = local write "当前状态："("Ready" ("当前状态：")) -> ()
          }
        }
        n194 = global read "device variables.vi" "VAR stop all"() -> (w336:bool)
      }
      n195 = local write "刷新设置"(TRUE ("刷新设置")) -> ()
      n196 = global write "device variables.vi" "VAR stop all"(w16) -> ()
      n197 = global write "device variables.vi" "VAR write data"(w12) -> ()
      n198 = property on="com-write" class="Bool (严格)"("Value"=w12) -> ()  [unwired: 2 in, 2 out]
      n199 = global write "device variables.vi" "VAR init"(w16) -> ()
      n200 = call <vilib>:"VISA Configure Serial Port (Instr).vi"("VISA resource name"="Port", "Enable Termination\nChar (T)"=TRUE ("Enable Termination\nChar (T)"), "baud rate (9600)"=u32 19200, "data bits (8)"=u16 8, "parity (0:none)"=enum16{"None", "Odd", "Even", "Mark", "Space"}."None", "stop bits (10: 1 bit)"=w32, "flow control (0:none)"=w13) -> ("VISA resource name out"=w9:refnum<visa-resource-name>, "error out"=w21:errorcluster)  [unwired: 7 in]
      n201 = register-events("dc level 1 in", "dc level 2 in", "dc level 3 in", "loop 1 in", "loop 2 in", "loop 3 in", "command in") -> (reference out=w38:refnum<event-registration>, error out=w27:errorcluster)  [unwired: 2 in]
      n202 = global write "device variables.vi" "VAR USB"(w9) -> ()
      n203 = VISA Open(error in (no error)=w21, VISA resource name=w9) -> (VISA resource name=w22:refnum<visa-resource-name>, error out=w23:errorcluster)  [unwired: 3 in]
      n204 = control-ref of="start sequence"() -> (w5:refnum<vi>)
      n205 = control-ref of="sequence string"() -> (w4:refnum<vi>)
      n206 = VISA Flush I/O Buffer(VISA resource name=w22, error in (no error)=w23) -> (VISA resource name out=w6:refnum<visa-resource-name>, error out=w7:errorcluster)  [unwired: 1 in]
      n207 = call "read data.vi"("VISA resource name in"=w6, "String End"="[\\r>]", "error in"=w7) -> ("error ende"=w14:errorcluster)  [unwired: 7 in]
      n208 = call "error.vi"("error 1"=w14) -> ()  [unwired: 11 in]
      n209 = call "refresh.vi"("error in"=w7, "VISA-Ressourcen-Name (In)"=w6, "reset all"=TRUE) -> ("init ok??"=w11:bool)  [unwired: 8 in]
      n210 = call "sequence.vi"("error in"=w7, "VISA-Ressourcen-Name"=w6, "Kommandozeilen Refnum"=w4, "Startbutton Refnum"=w5) -> ()  [unwired: 8 in]
      n211 = global write "device variables.vi" "VAR init"(w11) -> ()
      n212 = while {
        tunnel: w7 -> [w45]
        tunnel: w6 -> [w46]
        tunnel: w38 -> [w54]
        tunnel: w27 -> [w47]
        tunnel: [w53] -> w26
        tunnel: [w47] -> w25
        tunnel: [w50] -> w19
        tunnel: [w49] -> w18
        tunnel: [w48] -> w17
        stop <- w56 stop-if-true
        # "Eventschleife"
        n213 = event shown="[1] \"Drehschalter 0\", \"Drehschalter 1\", \"Drehschalter 2\": 值改变" {
          selector: w54 -> [_ _ _ _ _ _ _ _ _ _ _ _ _ _ _ _ _ _ _]
          dyn-events: [_ _ _ _ _ _ _ _ _ _ _ _ _ _ _ _ _ _ _] -> w53
          timeout: 500 -> [_ _ _ _ _ _ _ _ _ _ _ _ _ _ _ _ _ _ _]
          tunnel: [w65 w81 w94 w106 w121 w136 _ w148 w164 w181 w195 _ _ w214 _ w221 _ _ _] -> w59
          tunnel: [_ _ _ _ _ _ _ _ _ _ _ w208 _ _ _ _ _ _ _] -> w58
          tunnel: w46 -> [_ _ _ _ _ _ w147 _ _ _ _ _ _ _ _ _ _ _ _]
          tunnel: w45 -> [_ _ _ _ _ _ w146 _ _ _ _ _ _ _ _ _ _ _ _]
          tunnel: [FALSE _ _ _ _ TRUE _ TRUE TRUE TRUE TRUE _ _ TRUE _ TRUE _ _ _] -> w44
          event Timeout {
            # "bei timeout werte auslesen, wenn die initialisierung durch ist"
            n214 = global read "device variables.vi" "VAR init"() -> (w71:bool)
            n215 = global read "device variables.vi" "VAR device"() -> (w69:string)
            n216 = event-data() -> ()  [unwired: 1 in, 2 out]
            n217 = global read "device variables.vi" "VAR ver"() -> (w73:string)
            n218 = String Length(string=w73) -> (length=w72:i32)
            n219 = String Length(string=w69) -> (length=w70:i32)
            n220 = Greater Than 0?(x=w72) -> (x > 0?=w67:bool)
            n221 = Greater Than 0?(x=w70) -> (x > 0?=w68:bool)
            n222 = Concatenate Strings("measure" ("String"), "\r") -> (w62:string)
            n223 = Compound Arithmetic op=AND(w67, w71, w68) -> (w66:bool)
            n224 = Select(t=w62, s=w66, f="") -> (s? t:f=w65:string)
          }
          event "Drehschalter 0", "Drehschalter 1", "Drehschalter 2": Value Change {
            n225 = event-data() -> ("CtlRef"=w80:refnum<vi>)  [unwired: 1 in, 3 out]
            n226 = property class="Knob (严格)"(reference=w80) -> ("Value"=w76:dbl, "Label.Text"=w79:string)  [unwired: 1 in, 2 out]
            n227 = Number To Fractional String(use system decimal point (T)=FALSE ("Systemdezimalzeichen verwenden (T)"), number=w76, width (-)=i16 2 ("Breite (-)"), precision (6)=i16 3 ("Genauigkeit (6)")) -> (F-format string=w77:string)
            n228 = global write "device variables.vi" "VAR actualisation"(FALSE ("VAR mode changed")) -> ()
            n229 = Scan From String(format string="%s %d" ("Format-String"), input string=w79) -> (output 2=w75:i32)  [unwired: 5 in, 3 out]
            n230 = Format Into String(format string="%d,%s\r", initial string="set,", w75, w77) -> (resulting string=w81:string)  [unwired: 1 in, 1 out]
          }
          event Value Change {
            w88 = u8 0 ("Eingang 1")
            n231 = event-data() -> ("CtlRef"=w101:refnum<vi>)  [unwired: 1 in, 3 out]
            n232 = global read "device variables.vi" "Array dc-level"() -> (w90:dbl[])
            n233 = property class="Knob"(reference=w101) -> (error out=w93:errorcluster, "Value"=w92:variant)  [unwired: 1 in, 1 out]
            n234 = Variant To Data(error in=w93, type=0.0, Variant=w92) -> (data=w87:dbl)  [unwired: 1 out]
            n235 = Number To Fractional String(use system decimal point (T)=FALSE ("Systemdezimalzeichen verwenden (T)"), number=w87, width (-)=i16 2 ("Breite (-)"), precision (6)=i16 3 ("Genauigkeit (6)")) -> (F-format string=w95:string)
            n236 = Format Into String(format string="%d,%s\r", initial string="set,", w88, w95) -> (resulting string=w94:string)  [unwired: 1 in, 1 out]
            n237 = Replace Array Subset(array=w90, new element=w87, index=w88) -> (w89:dbl[])
            n238 = global write "device variables.vi" "Array dc-level"(w89) -> ()
            n239 = property on="Drehschalter 0" class="Knob (严格)"("Value"=w87) -> ()  [unwired: 2 in, 2 out]
          }
          event Value Change {
            w103 = u8 1 ("Eingang 1")
            n240 = event-data() -> ("CtlRef"=w107:refnum<vi>)  [unwired: 1 in, 3 out]
            n241 = global read "device variables.vi" "Array dc-level"() -> (w105:dbl[])
            n242 = property class="Knob"(reference=w107) -> (error out=w110:errorcluster, "Value"=w109:variant)  [unwired: 1 in, 1 out]
            n243 = Variant To Data(error in=w110, type=0.0, Variant=w109) -> (data=w102:dbl)  [unwired: 1 out]
            n244 = Number To Fractional String(use system decimal point (T)=FALSE ("Systemdezimalzeichen verwenden (T)"), number=w102, width (-)=i16 2 ("Breite (-)"), precision (6)=i16 3 ("Genauigkeit (6)")) -> (F-format string=w111:string)
            n245 = Format Into String(format string="%d,%s\r", initial string="set,", w103, w111) -> (resulting string=w106:string)  [unwired: 1 in, 1 out]
            n246 = Replace Array Subset(array=w105, new element=w102, index=w103) -> (w104:dbl[])
            n247 = global write "device variables.vi" "Array dc-level"(w104) -> ()
            n248 = property on="Drehschalter 1" class="Knob (严格)"("Value"=w102) -> ()  [unwired: 2 in, 2 out]
          }
          event Value Change {
            w118 = u8 2 ("Eingang 1")
            n249 = event-data() -> ("CtlRef"=w122:refnum<vi>)  [unwired: 1 in, 3 out]
            n250 = global read "device variables.vi" "Array dc-level"() -> (w120:dbl[])
            n251 = property class="Knob"(reference=w122) -> (error out=w125:errorcluster, "Value"=w124:variant)  [unwired: 1 in, 1 out]
            n252 = Variant To Data(error in=w125, type=0.0, Variant=w124) -> (data=w117:dbl)  [unwired: 1 out]
            n253 = Number To Fractional String(use system decimal point (T)=FALSE ("Systemdezimalzeichen verwenden (T)"), number=w117, width (-)=i16 2 ("Breite (-)"), precision (6)=i16 3 ("Genauigkeit (6)")) -> (F-format string=w126:string)
            n254 = Format Into String(format string="%d,%s\r", initial string="set,", w118, w126) -> (resulting string=w121:string)  [unwired: 1 in, 1 out]
            n255 = Replace Array Subset(array=w120, new element=w117, index=w118) -> (w119:dbl[])
            n256 = global write "device variables.vi" "Array dc-level"(w119) -> ()
            n257 = property on="Drehschalter 2" class="Knob (严格)"("Value"=w117) -> ()  [unwired: 2 in, 2 out]
          }
          event "Remote 0", "Remote 1", "Remote 2": Value Change {
            n258 = event-data() -> ("CtlRef"=w141:refnum<vi>, "NewVal"=w133:bool)  [unwired: 1 in, 4 out]
            n259 = global read "device variables.vi" "Array remote"() -> (w142:bool[])
            n260 = Boolean To (0,1)(Boolean=w133) -> (0, 1=w137:i16)
            n261 = property class="Bool (严格)"(reference=w141) -> ("Label.Text"=w134:string)  [unwired: 1 in, 2 out]
            n262 = Scan From String(format string="%s %d" ("Format-String"), input string=w134) -> (output 2=w135:i32)  [unwired: 5 in, 3 out]
            n263 = Replace Array Subset(array=w142, new element=w133, index=w135) -> (w143:bool[])
            n264 = global write "device variables.vi" "Array remote"(w143) -> ()
            n265 = Format Into String(format string="%d,%d\r" ("Format-String"), initial string="setk,", w135, w137) -> (resulting string=w136:string)  [unwired: 1 in, 1 out]
          }
          event "Refresh": Mouse Up {
            w145 = FALSE ("VAR init")
            # "refresh button gedrückt\n- variablen zurück setzen\n- keine messwerte abfragen"
            n266 = event-data() -> ()  [unwired: 1 in, 4 out]
            n267 = global write "device variables.vi" "VAR init"(w145) -> ()
            n268 = call "refresh.vi"("error in"=w146, "VISA-Ressourcen-Name (In)"=w147, "reset all"=w145) -> ("init ok??"=w144:bool)  [unwired: 8 in]
            n269 = global write "device variables.vi" "VAR init"(w144) -> ()
          }
          event "Loop 0", "Loop 1", "Loop 2": Value Change {
            # "Namen nicht ändern,\nsonst kommt die Abfrage\ndurcheinander"
            n270 = event-data() -> ("CtlRef"=w154:refnum<vi>, "NewVal"=w153:bool)  [unwired: 1 in, 4 out]
            n271 = property class="Bool (严格)"(reference=w154) -> ("Label.Text"=w152:string)  [unwired: 1 in, 2 out]
            n272 = global read "device variables.vi" "Array loop"() -> (w159:bool[])
            n273 = Boolean To (0,1)(Boolean=w153) -> (0, 1=w155:i16)
            n274 = Scan From String(format string="%s %d" ("Format-String"), input string=w152) -> (output 2=w151:i32)  [unwired: 5 in, 3 out]
            n275 = Replace Array Subset(array=w159, new element=w153, index=w151) -> (w160:bool[])
            n276 = global write "device variables.vi" "Array loop"(w160) -> ()
            n277 = Format Into String(format string="%d,%d\r" ("Format-String"), initial string="cloop,", w151, w155) -> (resulting string=w148:string)  [unwired: 1 in, 1 out]
            n278 = global write "device variables.vi" "VAR actualisation"(TRUE ("VAR mode changed")) -> ()
          }
          event Value Change {
            w162 = 0 ("Index")
            n279 = event-data() -> ("NewVal"=w163:bool)  [unwired: 1 in, 5 out]
            n280 = global read "device variables.vi" "Array IsActor"() -> (w166:bool[])
            n281 = Index Array(array=w166, index=w162) -> (element=w165:bool)
            n282 = case shown="真" w165 {
              tunnel: ["" w173] -> w164
              tunnel: w163 -> [_ w168]
              tunnel: w162 -> [_ w170]
              frame False {
              }
              frame True {
                n283 = global read "device variables.vi" "Array loop"() -> (w172:bool[])
                n284 = Replace Array Subset(array=w172, new element=w168, index=w170) -> (w171:bool[])
                n285 = Boolean To (0,1)(Boolean=w168) -> (0, 1=w169:i16)
                n286 = global write "device variables.vi" "Array loop"(w171) -> ()
                n287 = Format Into String(format string="%d\r" ("Format-String"), initial string="cloop,0," ("Anfangsstring"), w169) -> (resulting string=w173:string)  [unwired: 1 in, 1 out]
              }
            }
          }
          event Value Change {
            w177 = 1
            n288 = event-data() -> ("NewVal"=w178:bool)  [unwired: 1 in, 5 out]
            n289 = global read "device variables.vi" "Array IsActor"() -> (w180:bool[])
            n290 = Index Array(array=w180, index=w177) -> (element=w179:bool)
            n291 = case shown="真" w179 {
              tunnel: ["" w188] -> w181
              tunnel: w178 -> [_ w183]
              tunnel: w177 -> [_ w185]
              frame False {
              }
              frame True {
                n292 = global read "device variables.vi" "Array loop"() -> (w187:bool[])
                n293 = Replace Array Subset(array=w187, new element=w183, index=w185) -> (w186:bool[])
                n294 = Boolean To (0,1)(Boolean=w183) -> (0, 1=w184:i16)
                n295 = global write "device variables.vi" "Array loop"(w186) -> ()
                n296 = Format Into String(format string="%d\r" ("Format-String"), initial string="cloop,1," ("Anfangsstring"), w184) -> (resulting string=w188:string)  [unwired: 1 in, 1 out]
              }
            }
          }
          event Value Change {
            w192 = 2
            n297 = event-data() -> ("NewVal"=w193:bool)  [unwired: 1 in, 5 out]
            n298 = global read "device variables.vi" "Array IsActor"() -> (w196:bool[])
            n299 = Index Array(array=w196, index=w192) -> (element=w194:bool)
            n300 = case shown="真" w194 {
              tunnel: ["" w203] -> w195
              tunnel: w193 -> [_ w198]
              tunnel: w192 -> [_ w200]
              frame False {
              }
              frame True {
                n301 = global read "device variables.vi" "Array loop"() -> (w202:bool[])
                n302 = Replace Array Subset(array=w202, new element=w198, index=w200) -> (w201:bool[])
                n303 = Boolean To (0,1)(Boolean=w198) -> (0, 1=w199:i16)
                n304 = global write "device variables.vi" "Array loop"(w201) -> ()
                n305 = Format Into String(format string="%d\r" ("Format-String"), initial string="cloop,2," ("Anfangsstring"), w199) -> (resulting string=w203:string)  [unwired: 1 in, 1 out]
              }
            }
          }
          event "Stopp": Value Change {
            # "falls noch eine sequence läuft\ndann diese abbrechen"
            # "In der Hauptschleife wurde\ndie STOP Taste gedrückt"
            n306 = event-data() -> ("NewVal"=w209:bool)  [unwired: 1 in, 5 out]
            n307 = property on="start sequence" class="Bool (严格)"("Value"=FALSE ("start sequence")) -> ()  [unwired: 2 in, 2 out]
            n308 = Equal?(x=TRUE, y=w209) -> (x = y?=w208:bool)
          }
          event "Clear": Mouse Up {
            n309 = event-data() -> ()  [unwired: 1 in, 4 out]
            n310 = global write "device variables.vi" "Array Receive"(string[] [] ("Array Receive")) -> ()
            n311 = global write "device variables.vi" "Array Send"(string[] [] ("Array Send")) -> ()
          }
          event "Send": Mouse Up; "SendString": Value Change {
            # "prüfen ob Aktor angeschlossen ist"
            n312 = event-data() -> ()  [unwired: 1 in, 4 out]
            n313 = Concatenate Strings("SendString", "\r") -> (w215:string)
            n314 = call "test before send.vi"("data string in"=w215) -> ("send OK"=w216:bool)  [unwired: 10 in]
            n315 = Select(t=w215, s=w216, f="") -> (s? t:f=w214:string)
          }
          event "com-write": Value Change {
            # "mit schreiben der Daten im Fenster erlauben"
            n316 = event-data() -> ("NewVal"=w219:bool)  [unwired: 1 in, 5 out]
            n317 = global write "device variables.vi" "VAR write data"(w219) -> ()
          }
          event Value Change {
            # "prüfen, ob Aktor angeschlossen"
            # "Kommando wurde von aussen geschickt"
            n318 = event-data() -> ("NewVal"=w226:string)  [unwired: 1 in, 5 out]
            n319 = Concatenate Strings(w226, "\r") -> (w223:string)
            n320 = call "test before send.vi"("data string in"=w223) -> ("send OK"=w224:bool)  [unwired: 10 in]
            n321 = Select(t=w223, s=w224, f="") -> (s? t:f=w221:string)
          }
          event "start sequence": Value Change {
            n322 = event-data() -> ()  [unwired: 1 in, 6 out]
          }
          event "load sequence": Value Change {
            n323 = event-data() -> ("CtlRef"=w228:refnum<vi>)  [unwired: 1 in, 5 out]
            n324 = property class="Bool (严格)"(reference=w228, "Value"=FALSE ("Wert")) -> ()  [unwired: 1 in, 2 out]
            n325 = call "Dateidialog"("prompt"="Select the file to load", "pattern (all files)"="*.seq", "pattern label"="Sequence Files") -> ("selected path"=w234:path, "exists"=w230:bool, "error out"=w233:errorcluster)  [unwired: 9 in, 1 out]
            n326 = case shown="真" w230 {
              tunnel: w234 -> [_ w248]
              tunnel: w233 -> [_ w247]
              tunnel: T5."open" ("Operation (0:Öffnen)") -> [_ w245]
              tunnel: enum16{"read/write", "read-only", "write-only"}."read-only" ("Zugriff (0:Lesen/Schreiben)") -> [_ w244]
              tunnel: [w238 w239] -> w229
              frame False {
                (unwired) ""
                n327 = property on="sequence string" class="Str"() -> ("Text.Text"=w238:string)  [unwired: 2 in, 2 out]
              }
              frame True {
                n328 = Open/Create/Replace File(file path (use dialog)=w248, error in=w247, operation (0:open)=w245, access (0:read/write)=w244) -> (refnum out=w241:refnum<file>, error out=w240:errorcluster)  [unwired: 2 in, 1 out]
                n329 = Read from Text File(file (use dialog)=w241, error in=w240) -> (refnum out=w242:refnum<file>, text=w239:string, error out=w243:errorcluster)  [unwired: 2 in, 1 out]
                n330 = Close File(refnum=w242, error in=w243) -> (error out=w246:errorcluster)  [unwired: 1 out]
                n331 = call <vilib>:"Simple Error Handler.vi"("error in (no error)"=w246) -> ()  [unwired: 4 in, 5 out]
              }
            }
            n332 = property on="sequence string" class="Str"("Text.Text"=w229) -> ()  [unwired: 2 in, 2 out]
          }
          event "save sequence": Value Change {
            n333 = event-data() -> ("CtlRef"=w251:refnum<vi>)  [unwired: 1 in, 5 out]
            n334 = property class="Bool (严格)"(reference=w251, "Value"=FALSE ("Wert")) -> ()  [unwired: 1 in, 2 out]
            n335 = property on="sequence string" class="Str"() -> ("Text.Text"=w254:string)  [unwired: 2 in, 2 out]
            n336 = call "Dateidialog2"("prompt"="Select the file to save", "pattern (all files)"="*.seq", "pattern label"="Sequence Files") -> ("selected path"=w256:path, "cancelled"=w249:bool, "error out"=w255:errorcluster)  [unwired: 9 in, 1 out]
            n337 = case shown="真" w249 {
              tunnel: w256 -> [w269 _]
              tunnel: w255 -> [w268 _]
              tunnel: w254 -> [w267 _]
              tunnel: T5."replace or create" ("Operation (0:Öffnen)") -> [w266 _]
              tunnel: enum16{"read/write", "read-only", "write-only"}."write-only" ("Zugriff (0:Lesen/Schreiben)") -> [w265 _]
              frame False {
                n338 = Open/Create/Replace File(file path (use dialog)=w269, error in=w268, operation (0:open)=w266, access (0:read/write)=w265) -> (refnum out=w264:refnum<file>, error out=w261:errorcluster)  [unwired: 2 in, 1 out]
                n339 = Write to Text File(file (use dialog)=w264, text=w267, error in=w261) -> (refnum out=w262:refnum<file>, error out=w263:errorcluster)  [unwired: 1 in, 1 out]
                n340 = Close File(refnum=w262, error in=w263) -> (error out=w260:errorcluster)  [unwired: 1 out]
                n341 = call <vilib>:"Simple Error Handler.vi"("error in (no error)"=w260) -> ()  [unwired: 4 in, 5 out]
              }
              frame True {
              }
            }
          }
        }
        n342 = global read "device variables.vi" "VAR stop all"() -> (w57:bool)
        n343 = call "senddata.vi"("read ERR"=w44, "error in"=w45, "writebuffer"=w59, "VISA-Ressourcen-Name"=w46) -> ("error out"=w51:errorcluster, "VISA-Ressourcen-Name (Ausgang)"=w52:refnum<visa-resource-name>)  [unwired: 5 in, 1 out]
        n344 = Or(x=w58, y=w57) -> (x .or. y?=w56:bool)
        n345 = property class="Instr"(reference=w52, error in=w51) -> (reference out=w50:refnum<visa-resource-name>, error out=w49:errorcluster, "Is Connected"=w48:bool)
      }
      n346 = while {
        stop <- "Stopp" stop-if-true
        # "程序运行期间部分功能不可用"
        # "如果太大，那么\n删除最后一项"
        # "更新显示"
        # "自定义设置页面按钮"
        # "设置旋转开关的值"
        n347 = global read "device variables.vi" "Array dc-level closed"() -> (w281:dbl[])
        n348 = global read "device variables.vi" "Array dc-level open"() -> (w282:dbl[])
        n349 = global read "device variables.vi" "Array actor-name"() -> (w323:string[])
        n350 = global read "device variables.vi" "VAR actualisation"() -> (w279:bool)
        n351 = control-ref of="Registerkarte"() -> (w277:refnum<vi>)
        n352 = global read "device variables.vi" "Array dc-level"() -> (w320:dbl[])
        n353 = global read "device variables.vi" "Array IsActor"() -> (w301:bool[])
        n354 = global read "device variables.vi" "Array remote"() -> (w278:bool[])
        n355 = global read "device variables.vi" "Array clmax"() -> (w308:dbl[])
        n356 = global read "device variables.vi" "Array clmin"() -> (w309:dbl[])
        n357 = global read "device variables.vi" "VAR Temp"() -> (w325:string)
        n358 = global read "device variables.vi" "Array loop"() -> (w300:bool[])
        n359 = global read "device variables.vi" "VAR Vmax"() -> (w306:dbl)
        n360 = global read "device variables.vi" "Array axis"() -> (w322:string[])
        n361 = global read "device variables.vi" "VAR Vmin"() -> (w307:dbl)
        n362 = global read "device variables.vi" "Array ovl"() -> (w321:bool[])
        n363 = global read "device variables.vi" "VAR USB"() -> (w324:string)
        n364 = control-ref of="Drehschalter 0"() -> (w305:refnum<vi>)
        n365 = control-ref of="Drehschalter 1"() -> (w304:refnum<vi>)
        n366 = control-ref of="Drehschalter 2"() -> (w303:refnum<vi>)
        n367 = Index Array(array=w320) -> (element #1=w319:dbl, element #2=w318:dbl, element #3=w317:dbl)  [unwired: 3 in]
        n368 = Bundle("Registerkarte"=w277, "Array IsActor"=w301, "Array loop"=w300, "Array remote"=w278) -> (w276:T6)  [unwired: 1 in]
        n369 = Bundle("Array dc-level"=w320, "VAR Temp"=w325, "VAR USB"=w324, "Array IsActor"=w301, "Array actor-name"=w323, "Array axis"=w322, "Array loop"=w300, "Array remote"=w278, "Array ovl"=w321) -> (w302:T7)  [unwired: 1 in]
        n370 = Bundle("Drehschalter 0"=w305, "Drehschalter 1"=w304, "Drehschalter 2"=w303, "Array loop"=w300, "Array IsActor"=w301, "Array clmin"=w309, "Array clmax"=w308, "VAR Vmin"=w307, "VAR Vmax"=w306, "Array dc-level open"=w282, "Array dc-level closed"=w281, "VAR actualisation"=w279) -> (w280:T8)  [unwired: 1 in]
        n371 = call "set buttons.vi"("Cluster Button"=w276) -> ()  [unwired: 11 in]
        n372 = call "set controller.vi"("Cluster Controller"=w280) -> ()  [unwired: 12 in, 3 out]
        n373 = call "display.vi"("Cluster Display In"=w302) -> ("Display - Refnum"=w326:refnum<vi>)  [unwired: 10 in]
        n374 = invoke on="Unterpanel1" class="SubPnl" method="Insert VI"("VI Ref"=w326) -> ()  [unwired: 3 in, 4 out]
        n375 = property class="DigNum"(reference="dc level 1 out", "Value"=w319) -> (error out=w316:errorcluster)  [unwired: 1 in, 1 out]
        n376 = property class="DigNum"(reference="dc level 2 out", "Value"=w318) -> (error out=w315:errorcluster)  [unwired: 1 in, 1 out]
        n377 = property class="DigNum"(reference="dc level 3 out", "Value"=w317) -> (error out=w314:errorcluster)  [unwired: 1 in, 1 out]
        n378 = global read "device variables.vi" "VAR max array"() -> (w291:i32)
        n379 = global read "device variables.vi" "Array Receive"() -> (w290:string[])
        n380 = call "error.vi"("error 5"=w316, "error 2"=w314, "error 1"=w315) -> ()  [unwired: 9 in]
        n381 = global read "device variables.vi" "Array Send"() -> (w289:string[])
        n382 = property on="start sequence" class="Bool (严格)"() -> ("Value"=w273:bool)  [unwired: 2 in, 2 out]
        n383 = global read "device variables.vi" "VAR last command"() -> (→"Last Command":string)
        n384 = global read "device variables.vi" "VAR last error"() -> (→"Last Error":string)
        n385 = global read "device variables.vi" "VAR device"() -> (→"Device":string)
        n386 = global read "device variables.vi" "VAR serno"() -> (→"Serial Number":string)
        n387 = global read "device variables.vi" "VAR date"() -> (→"Firmware Release Date":string)
        n388 = global read "device variables.vi" "VAR ver"() -> (→"Version Number":string)
        n389 = Array Size(array=w289) -> (size(s)=w288:i32)
        n390 = Array Size(array=w290) -> (size(s)=w285:i32)
        n391 = Select(t=u8 2 ("Deaktiviert"), s=w273, f=u8 0) -> (s? t:f=w272:u8)
        n392 = Greater Or Equal?(x=w288, y=w291) -> (x >= y?=w287:bool)
        n393 = Greater Or Equal?(x=w285, y=w291) -> (x >= y?=w286:bool)
        n394 = case shown="真" w287 {
          tunnel: [w328 w329] -> w283
          tunnel: w289 -> [w328 w331]
          tunnel: w291 -> [_ w330]
          frame False {
          }
          frame True {
            n395 = Delete From Array(array=w331, index=w330) -> (array with subset deleted=w329:string[])  [unwired: 1 in, 1 out]
            n396 = global write "device variables.vi" "Array Send"(w329) -> ()
          }
        }
        n397 = case shown="真" w286 {
          tunnel: w291 -> [_ w335]
          tunnel: [w332 w333] -> w284
          tunnel: w290 -> [w332 w334]
          frame False {
          }
          frame True {
            n398 = Delete From Array(array=w334, index=w335) -> (array with subset deleted=w333:string[])  [unwired: 1 in, 1 out]
            n399 = global write "device variables.vi" "Array Receive"(w333) -> ()
          }
        }
        n400 = property on="load sequence" class="Bool (严格)"("Disabled"=w272) -> ()  [unwired: 2 in, 2 out]
        n401 = property on="save sequence" class="Bool (严格)"("Disabled"=w272) -> ()  [unwired: 2 in, 2 out]
        n402 = property on="sequence string" class="Str"("Disabled"=w272) -> ()  [unwired: 2 in, 2 out]
        n403 = Wait (ms)(milliseconds to wait=u32 20 ("Zu wartende ms")) -> ()  [unwired: 1 out]
        n404 = global write "device variables.vi" "VAR stop all"("Stopp") -> ()
        n405 = Array To Spreadsheet String(array=w283, 3:"%s" ("Format-String")) -> (spreadsheet string=→"Send Buffer":string)  [unwired: 1 in]
        n406 = Array To Spreadsheet String(array=w284, 3:"%s" ("Format-String")) -> (spreadsheet string=→"Receive Buffer":string)  [unwired: 1 in]
      }
      n407 = Unregister For Events(event registration refnum=w26, error in=w25) -> (error out=w24:errorcluster)
      n408 = case shown="真" w17 {
        tunnel: w19 -> [_ w43]
        tunnel: w18 -> [_ w42]
        frame False {
        }
        frame True {
          n409 = VISA Close(VISA resource name=w43, error in (no error)=w42) -> (error out=w41:errorcluster)
          n410 = call "error.vi"("error 4"=w41) -> ()  [unwired: 11 in]
        }
      }
      n411 = call "error.vi"("error 4"=w24) -> ()  [unwired: 11 in]
    }
  }
